vi "Gaussian Noise.vi"(0 "image in":refnum<class "MSC Image.lvclass">, 1 "Mean":dbl=128.0, 2 "Std Dev":dbl=31.0, 5 "error in (no error)":errorcluster) -> (14 "image out":refnum<class "MSC Image.lvclass">, 19 "error out":errorcluster)   [LabVIEW 2014, in "MSC Image.lvclass"]
doc: "Replaces the image with gaussian noise."
uses:
  MSC Image.lvclass
  MSC Image.lvclass/MSC Image.ctl
  Dependencies/x86/MSC I Process32.dll
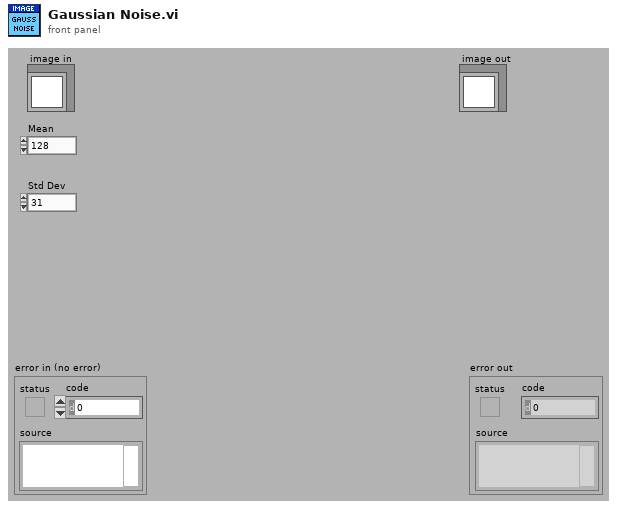
[diagram p1: front panel]
types:
  T1 = typedef "Image.ctl" = cluster{"Pointer":u64, "Size":T2, "Image Type":T3, "Time Stamp":timestamp, "Variant":variant}
  T2 = typedef "Size.ctl" = cluster{"Cols":i32, "Rows":i32}
  T3 = typedef "Image Type.ctl" = i32
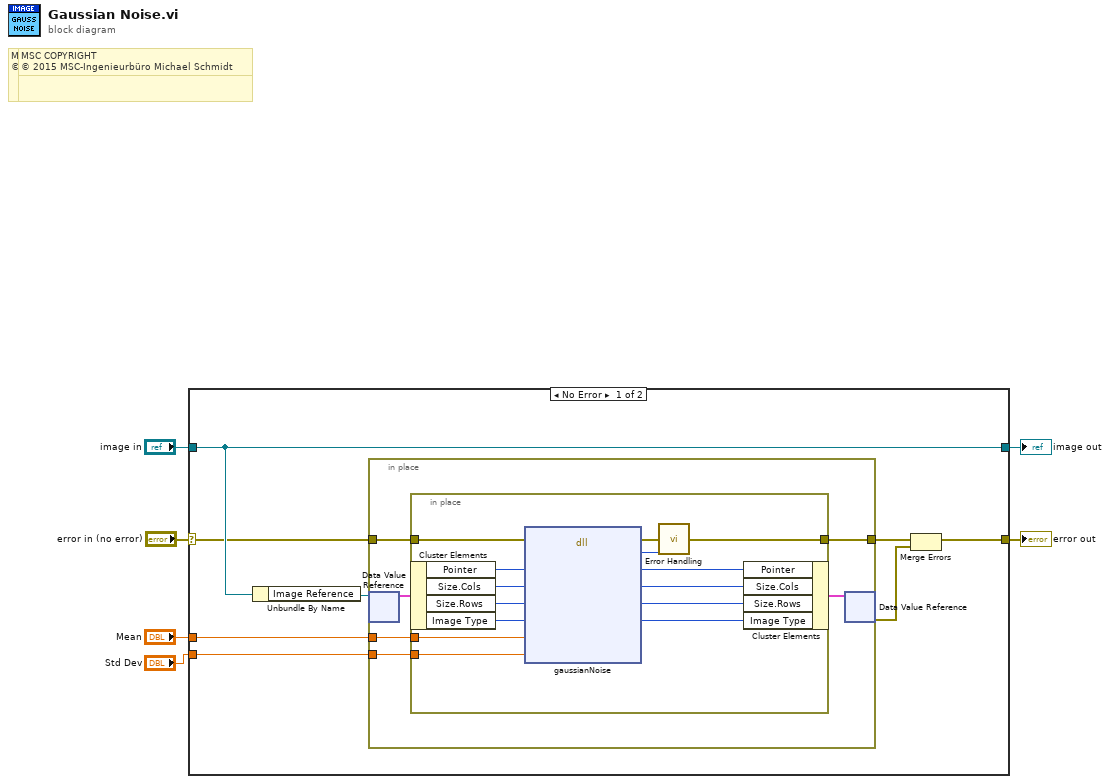
[diagram p0: block diagram]
diagram:
  # "MSC COPYRIGHT\n© 2016 MSC-Ingenieurbüro Michael Schmidt"
  # "MSC COPYRIGHT\n© 2016 MSC-Ingenieurbüro Michael Schmidt"
  # "MSC COPYRIGHT\n© 2015 MSC-Ingenieurbüro Michael Schmidt"
  # "MSC COPYRIGHT\n© 2015 MSC-Ingenieurbüro Michael Schmidt"
  n1 = case shown="No Error" "error in (no error)" {
    selector: "error in (no error)" -> [w10 w36]
    tunnel: [w9 w36] -> w5
    tunnel: [w14 w35] -> w3
    tunnel: "image in" -> [w14 w35]
    tunnel: "Mean" -> [w8 _]
    tunnel: "Std Dev" -> [w7 _]
    frame No Error {
      n2 = Unbundle By Name(w14) -> ("Image Reference"=w13:refnum<data-value>)
      n3 = in-place {
        in-place-border: w10 -> [w18]
        in-place-border: [w17] -> w12
        in-place-border: w8 -> [w16]
        in-place-border: w7 -> [w15]
        n4 = in-place-dvr #1(w13) -> (w19:T1)  [unwired: 1 out]
        n5 = in-place {
          in-place-border: w18 -> [w23]
          in-place-border: [w34] -> w17
          in-place-border: w16 -> [w22]
          in-place-border: w15 -> [w21]
          n6 = in-place-cluster #2(w19) -> ("Pointer"=w24:u64, "Size.Cols"=w29:i32, "Size.Rows"=w28:i32, "Image Type"=w25:T3)
          n7 = dll-call lib="C:/Users/MSC/LabVIEW Projekte/LV 2014/MSC I-Process/user.lib/MSC-I Process/Dependencies/x86/MSC I Process*.dll" fn="gaussianNoise"(error in=w23, "pointer"=w24, "cols"=w29, "rows"=w28, "type"=w25, "mean"=w22, "stdDev"=w21) -> (error out=w33:errorcluster, "error"=w32:i32, "pointer"=w31:u64, "cols"=w30:i32, "rows"=w27:i32, "type"=w26:i32)  [unwired: 4 in, 1 out]
          n8 = call "Error Handling.vi"("error in (no error)"=w33, "return type"=w32) -> ("error out"=w34:errorcluster)  [unwired: 12 in, 1 out]
          n9 = in-place-cluster #2("Pointer"=w31, "Size.Cols"=w30, "Size.Rows"=w27, "Image Type"=w26) -> (w20:T1)
        }
        n10 = in-place-dvr #1(w20) -> (w11:errorcluster)  [unwired: 1 out]
      }
      n11 = Merge Errors(w12, w11) -> (w9:errorcluster)
    }
    frame Error {
    }
  }
  "error out" <- w5
  "image out" <- w3
